vi "Periodic Tasks.vi"(8 "error in":errorcluster) -> ()   [LabVIEW 2023]
doc: "This VI runs in parallel to other tasks. It can contain as many user-defined periodic loops as you need. These can carry out PID or other sorts of timed response."
uses:
  <vilib>/Rock Robotics/WPI/DriverStation/WPI_DriverStationAllianceInfo.ctl
  ctrl defs/ctrl DRIVING FRAME selector.ctl
  ctrl defs/ctrl pivot select.ctl
  ctrl defs/ctrl driver input.ctl
  ctrl defs/ctrl FRONT FACE selector.ctl
  ctrl defs/ctrl XY coord.ctl
  ctrl defs/ctrl DRIVER target assist.ctl
  ctrl defs/ctrl LIMELIGHT STREAM selector.ctl
  ctrl defs/ctrl LIMELIGHT CAMMODE selector.ctl
  ctrl defs/ctrl LIMELIGHT LEDMODE selector.ctl
  <vilib>/Analysis/coordinate.llb/Angle Units.ctl
  <vilib>/Analysis/coordinate.llb/Angle Range (Degree).ctl
  <vilib>/Analysis/coordinate.llb/Wrap Angle (scalar).vi
  Global odometry.vi
  Global INIT.vi
  <vilib>/Analysis/NI_AAL_Angle.lvlib
panel:
  out "LimeLIGHT control":T4 {"stream" items=["standard side-by-side", "PiP Main", "PiP Secondary"]; "camMode" items=["Vision processor", "Driver Camera"]; "ledMode" items=["default to current pipeline", "force off", "force blink", "force on"]}
  out "DRIVER TARGET ASSIST":T5={"ASSIST?"=FALSE, "LOCKED ON?"=FALSE, "DistanceToTarget (in)"=26.235051697949295, "BRNG (deg)"=-2.0}
  out "Continuous Angle":T6
  in  "Update":bool
  out "pivot center":T7 {"Y" format="%.4g"; "X" format="%.4g"}
  out "front face":T8
  out "DRIVER INPUT":T9 {"Jr" format="%.4g"; "theta (rad)" format="%_4f"; "R" format="%.4g"; "Jy" format="%.4g"; "theta (deg)" format="%_4f"; "Jx" format="%.4g"}
  out "select pivot point":T10
  out "drive frame":T11
  out "Alliance":T12
  out "STEER":dbl
  out "DRIVE":dbl
  out "YRPHfH":T13
  out "REAR RIGHT":dbl(knob)
  out "V RR":dbl(knob) scale=-1.0..1.0
  out "FRONT RIGHT":dbl(knob)
  out "V FR":dbl(knob) scale=-1.0..1.0
  out "REAR LEFT":dbl(knob)
  out "V RL":dbl(knob) scale=-1.0..1.0
  out "FRONT LEFT":dbl(knob)
  out "V FL":dbl(knob) scale=-1.0..1.0
  out "Magnetic\nHeadings":cluster{dbl, dbl, dbl}(knob)={0.0, 140.19422999815168, 0.0} scale=0.0..360.0
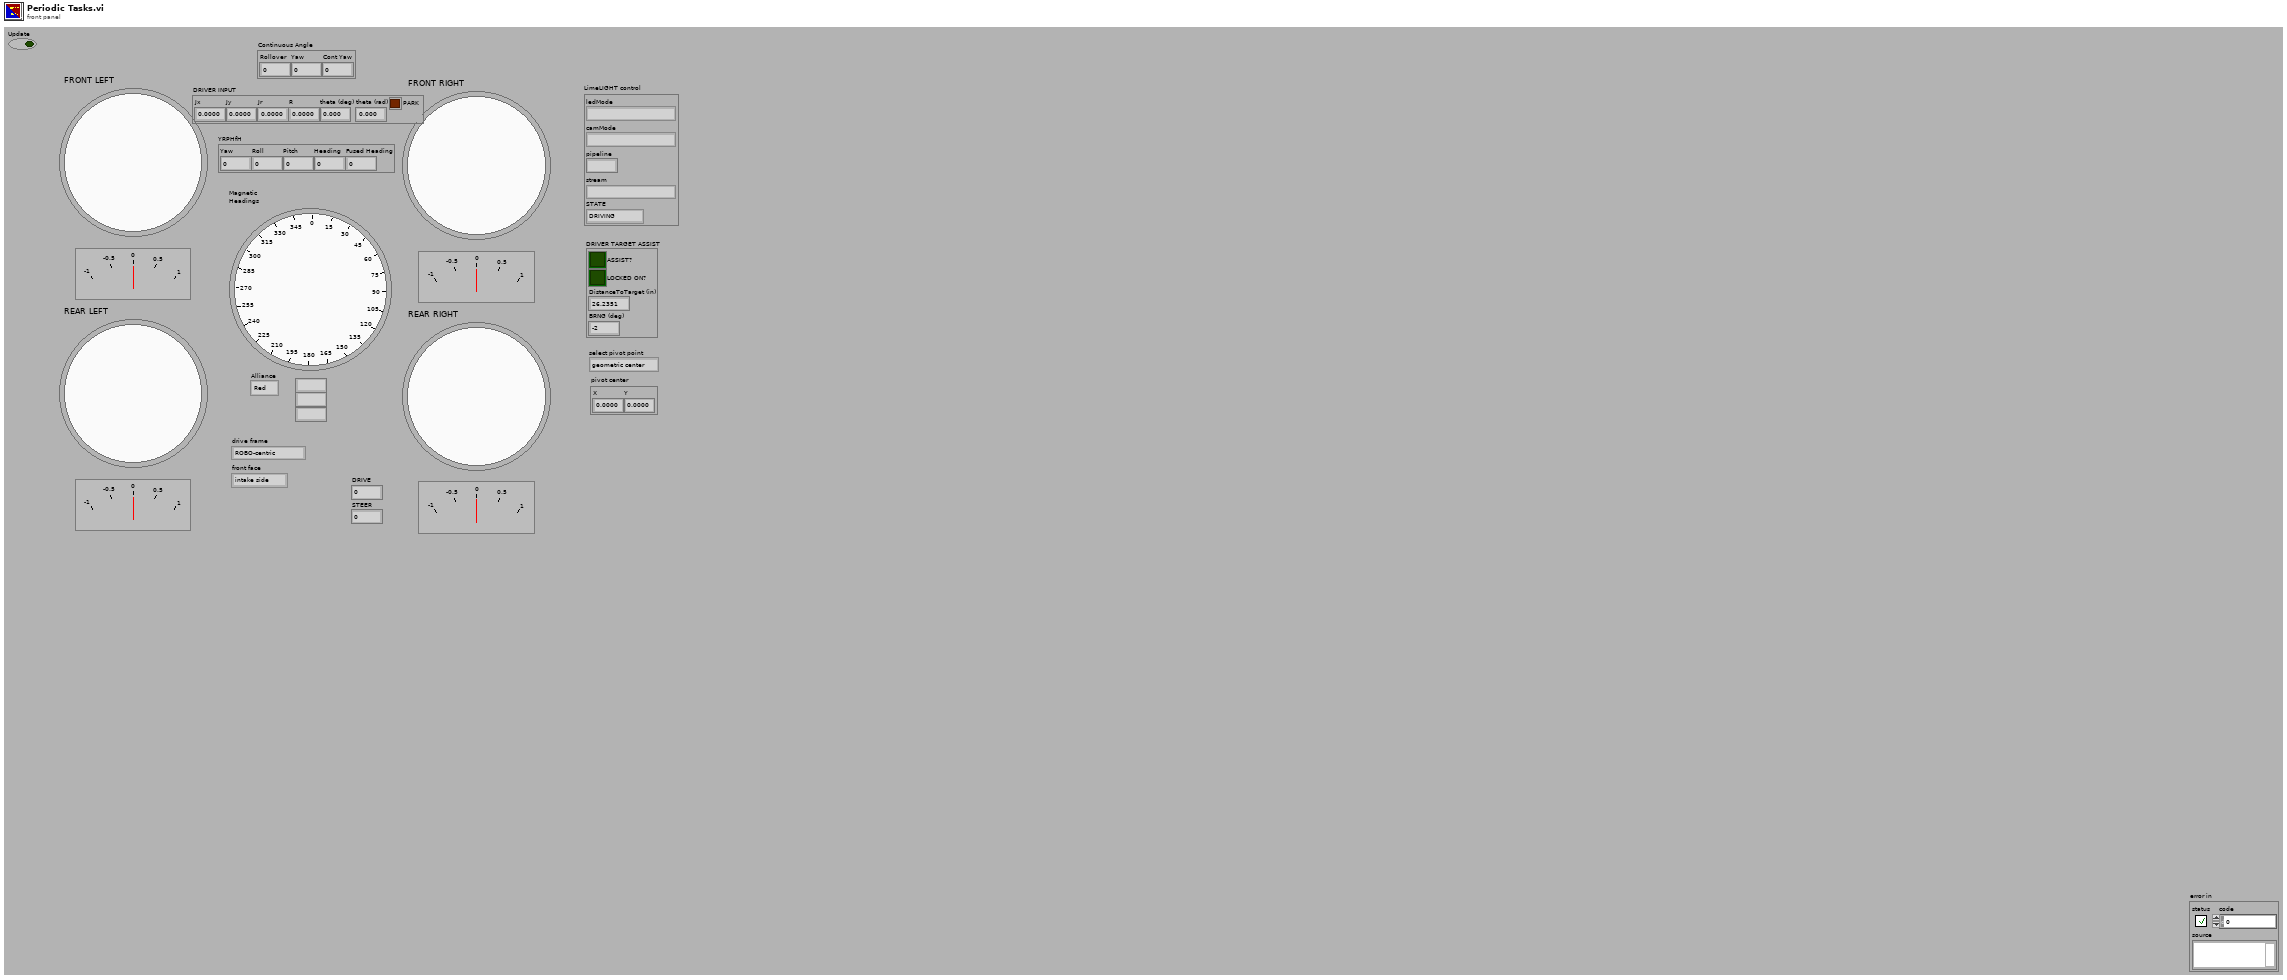
[diagram p1: front panel]
types:
  T1 = typedef "ctrl LIMELIGHT STREAM selector.ctl" = u16
  T2 = typedef "ctrl LIMELIGHT CAMMODE selector.ctl" = u16
  T3 = typedef "ctrl LIMELIGHT LEDMODE selector.ctl" = u16
  T4 = cluster{"stream":T1, "pipeline":u16, "camMode":T2, "ledMode":T3, "STATE":enum16{"DRIVING", "LOOKING for NOTE", "HAVE NOTE"}}
  T5 = typedef "ctrl DRIVER target assist.ctl" = cluster{"ASSIST?":bool, "LOCKED ON?":bool, "DistanceToTarget (in)":dbl, "BRNG (deg)":dbl}
  T6 = cluster{"Rollover":dbl, "Yaw":dbl, "Cont Yaw":dbl}
  T7 = typedef "ctrl XY coord.ctl" = cluster{"X":dbl, "Y":dbl}
  T8 = typedef "ctrl FRONT FACE selector.ctl" = enum16{"intake side", "shooter side"}
  T9 = typedef "ctrl driver input.ctl" = cluster{"Jx":dbl, "Jy":dbl, "Jr ":dbl, "R":dbl, "theta (deg)":dbl, "theta (rad)":dbl, "PARK":bool}
  T10 = typedef "ctrl pivot select.ctl" = enum16{"geometric center", "CG", "FL", "FR", "RR", "RL", "other"}
  T11 = typedef "ctrl DRIVING FRAME selector.ctl" = enum16{"ROBO-centric", "FLD-centric"}
  T12 = typedef "WPI_DriverStationAllianceInfo.ctl" = enum16{"Red", "Blue", "Invalid"}
  T13 = cluster{"Yaw":dbl, "Roll":dbl, "Pitch":dbl, "Heading":dbl, "Fused Heading":dbl}
  T14 = typedef "ctrl arm motor.ctl" = cluster{" motor":T15, "limit polarities":T21}
  T15 = typedef "ctrl swerve motor.ctl" = cluster{"description":string, "MOTOR SELECT":T16, "Installed?":bool, "CAN ID":u8, "refnum name":string, "Invert":bool, "Idle Mode":T17, "Current limiting":T18, "MOTOR PIDF coefficients":T19, "gear ratio":dbl}
  T16 = typedef "ctrl MOTOR SELECT.ctl" = i16
  T17 = typedef "Spark MAX Idle Mode.ctl" = enum16{"Coast", "Brake"}
  T18 = typedef "ctrl Spark MAX current limiting.ctl" = cluster{"Linearized":bool, "Free Speed (A)":dbl, "Primay (A)":dbl, "Limit RPM (0)":u32}
  T19 = typedef "ctrl motor PIDF coefficients.ctl" = cluster{"PIDF":cluster{"P Gain":dbl, "I Gain":dbl, "D Gain":dbl, "F Gain":dbl, "I Zone":dbl, "Min Output":dbl, "Max Output":dbl}, "Smart Motion":T20}
  T20 = typedef "Spark MAX Smart Motion Parameters.ctl" = cluster{"Max Velocity":dbl, "Max Acceleration":dbl, "Minimum Velocity Output":dbl, "Allowed Closed Loop Error":dbl}
  T21 = typedef "ctrl limit polarity.ctl" = cluster{"Forward limit":T22, "Reverse limit":T22}
  T22 = typedef "Spark MAX Limit Switch Polarity.ctl" = enum16{"Normally Open", "Normally Closed"}
  T23 = typedef "ctrl LED init.ctl" = cluster{"PWM Channel":T24, "refnum name":string, "#LEDS":T25, "initial output":dbl, "stack name":string, "Installed?":bool, "pattern":T26}
  T24 = typedef "FPGA_DIOPWMChannel.ctl" = enum8{"PWM 0", "PWM 1", "PWM 2", "PWM 3", "PWM 4", "PWM 5", "PWM 6", "PWM 7", "PWM 8", "PWM 9", "PWM MXP 0", "PWM MXP 1", "PWM MXP 2", "PWM MXP 3", "PWM MXP 4", "PWM MXP 5", "PWM MXP 6", "PWM MXP 7", "PWM MXP 8", "PWM MXP 9", "Invalid"}
  T25 = typedef "ctrl number of LEDs.ctl" = u16
  T26 = typedef "ctrl LED PATTERNS.ctl" = u16
  T27 = typedef "ctrl DIO.ctl" = cluster{"description":string, "Installed?":bool, "DIOChannel":T28, "refnum name":string}
  T28 = typedef "FPGA_DIOChannel.ctl" = enum8{"DIO 0", "DIO 1", "DIO 2", "DIO 3", "DIO 4", "DIO 5", "DIO 6", "DIO 7", "DIO 8", "DIO 9", "DIO MXP 0", "DIO MXP 1", "DIO MXP 2", "DIO MXP 3", "DIO MXP 4", "DIO MXP 5", "DIO MXP 6", "DIO MXP 7", "DIO MXP 8", "DIO MXP 9", "DIO MXP 10", "DIO MXP 11", "DIO MXP 12", "DIO MXP 13", "DIO MXP 14", "DIO MXP 15", "SPI Port CS1", "SPI Port CS2", "SPI Port CS3", "SPI Port MISO", "SPI Port MOSI", "Invalid"}
  T29 = typedef "ctrl LIMELIGHT initialize.ctl" = cluster{"Installed?":bool, "pose":cluster{"X":dbl, "Y":dbl, "Z":dbl, "angle to horizon":dbl, "tx angle offset":dbl}}
  T30 = typedef "WPI_DigitalInputDevRef.ctl" = cluster{"DevStatus":errorcluster, "DIO Channel":T28}
  T31 = typedef "ctrl swerve speeds.ctl" = cluster{"NORMAL":cluster{"DRIVE":dbl, "STEER":dbl}, "TURTLE":cluster{"DRIVE":dbl, "STEER":dbl}, "TURBO":cluster{"DRIVE":dbl, "STEER":dbl}}
  T32 = typedef "ctrl solenoid.ctl" = cluster{"description":string, "Installed?":bool, "refnum name":string, "coils":enum16{"Single", "Double"}, "forward channel":T33, "reverse channel":T33, "initial value":T34}
  T33 = typedef "WPI_SolenoidChannel.ctl" = enum8{"Solenoid 0", "Solenoid 1", "Solenoid 2", "Solenoid 3", "Solenoid 4", "Solenoid 5", "Solenoid 6", "Solenoid 7", "Solenoid 8", "Solenoid 9", "Solenoid 10", "Solenoid 11", "Solenoid 12", "Solenoid 13", "Solenoid 14", "Solenoid 15", "Invalid"}
  T34 = typedef "WPI_SolenoidValue.ctl" = enum16{"Off", "On", "Forward", "Reverse"}
  T35 = cluster{"LEFT ARM":cluster{"VBus%":dbl, "LOCK?":bool, "LOCKED":bool}, "RIGHT ARM":cluster{"VBus%":dbl, "LOCK?":bool, "LOCKED":bool}}
  T36 = cluster{"VBus%":dbl, "LOCK?":bool, "LOCKED":bool}
  T37 = typedef "WPI_MotorControlDeviceRef.ctl" = cluster{"DeviceStatus":errorcluster, "Type":T38, "PWM":cluster{"PWM Channel":T24, "DeadBand":T39}, "CAN":cluster{"Device Number":u8, "SetOutput VI Ref":variant, "GetOutput VI Ref":variant, "Enable VI Ref":variant, "Disable VI Ref":variant, "Data":variant}, "Invert":bool, "DIO PWM":cluster{"PWM \"Enable\" Channel":T24, "DIOChannel":T28, "PWM Rate":dbl}}
  T38 = typedef "WPI_MotorControlType.ctl" = enum16{"PWM", "CAN", "DIO PWM"}
  T39 = typedef "WPI_PWMDeadband.ctl" = cluster{"Name":string, "maxPositivePwm":i32, "minPositivePwm":i32, "centerPwm":i32, "maxNegativePwm":i32, "minNegativePwm":i32, "angularRange":u16}
  T40 = typedef "CTRE_Phoenix_CANcoder_DeviceRef.ctl" = cluster{"DeviceStatus":errorcluster, "Device Number":u8, "Handle":u64, "UsageFrame":u32, "Library Path":path}
  T41 = cluster{"Driver":T37, "Steer":T37, "Encoder":T40}[]
  T42 = typedef "NI_AAL_Angle.lvlib/Angle Range (Degree).ctl" = u16
  T43 = typedef "NI_AAL_Angle.lvlib/Angle Units.ctl" = i32
  T44 = cluster{"Heading":dbl, "MAGNETIC Zero for Blue Alliance (deg)":dbl, "angle out":dbl}
  T45 = typedef "ctrl DRIVER MODE.ctl" = enum16{"default", "TURTLE", "TURBO"}
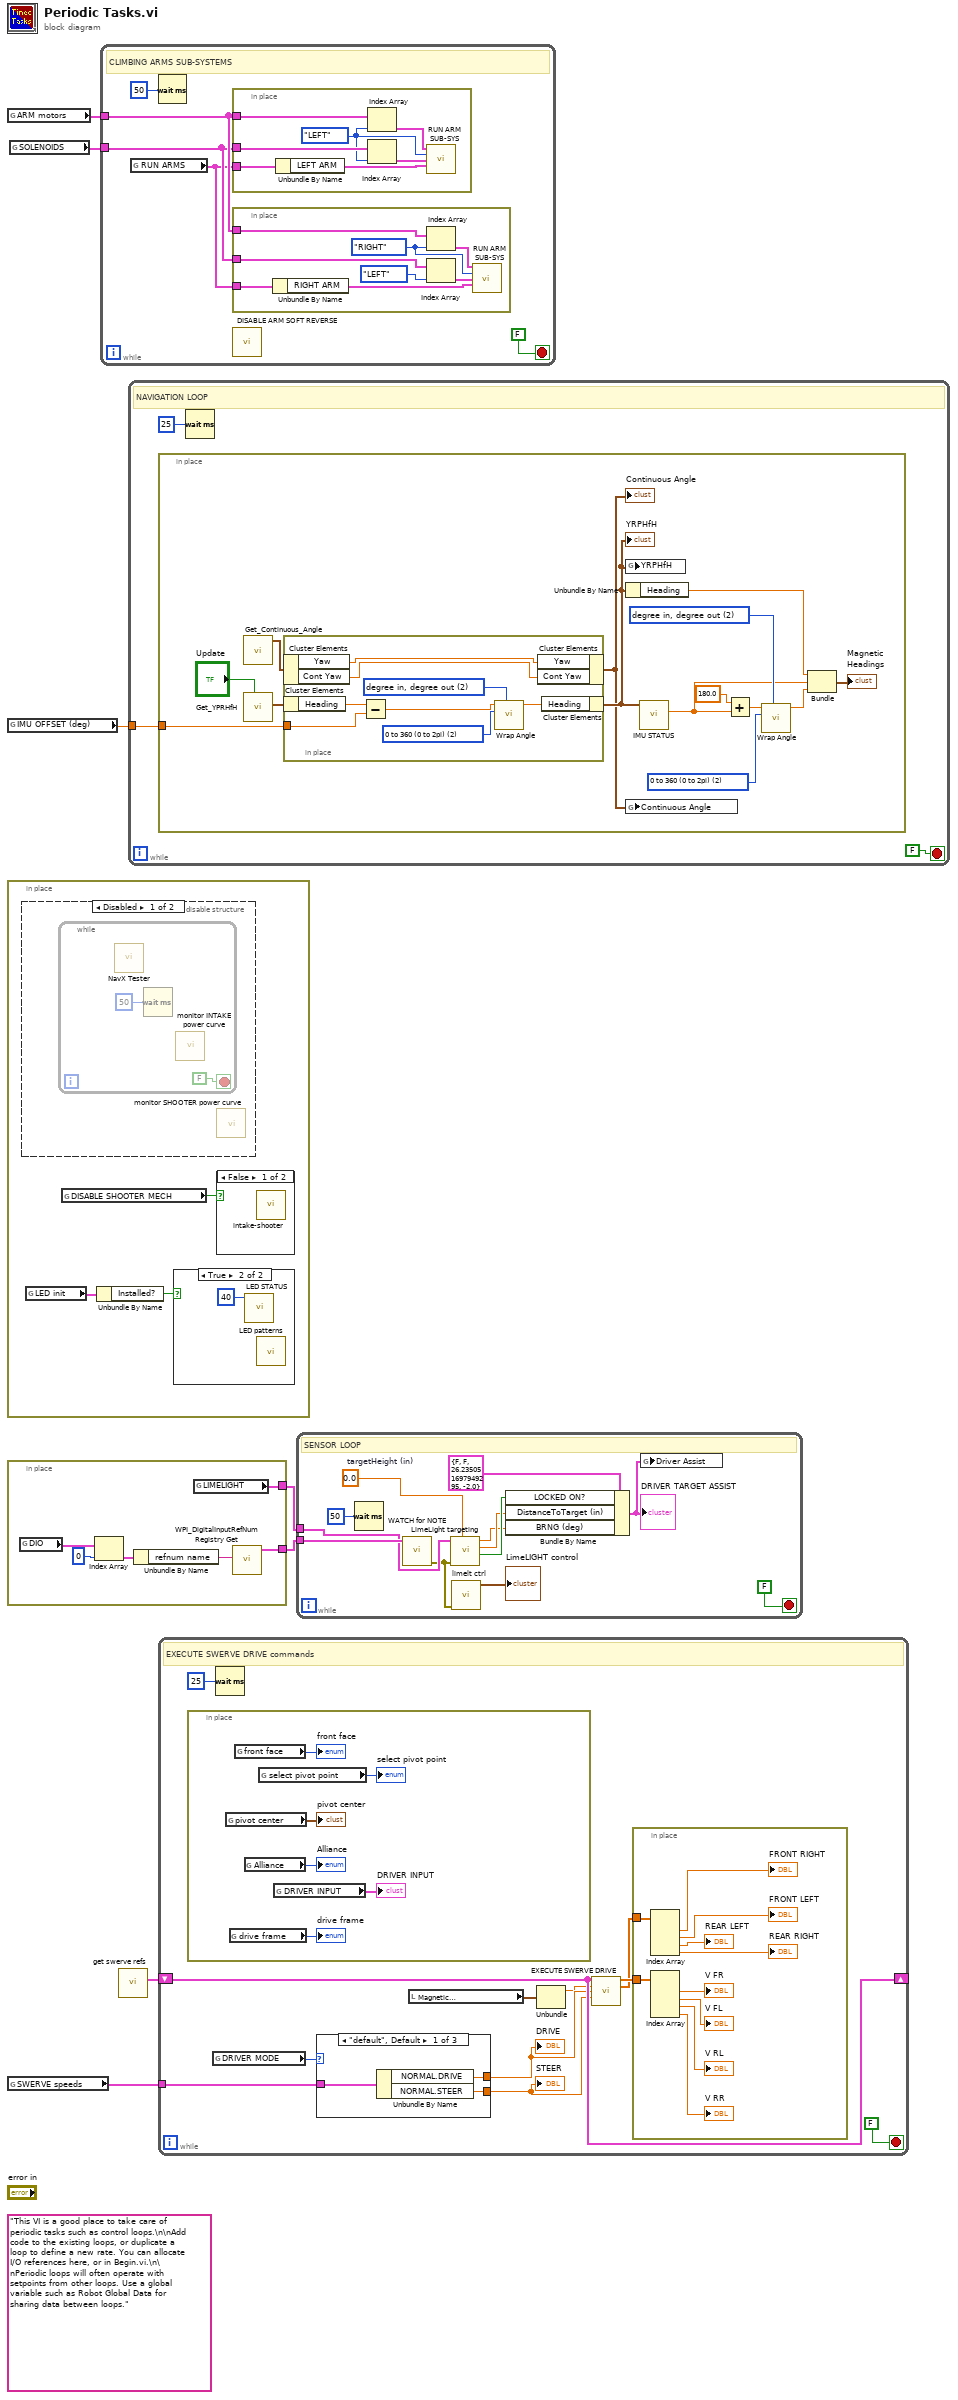
[diagram p0: block diagram]
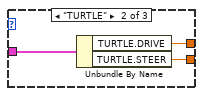
[diagram p5: hidden frame]
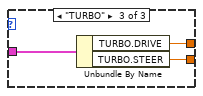
[diagram p6: hidden frame]
diagram:
  (unwired) "This VI is a good place to take care of periodic tasks such as control loops.\n\nAdd code to the existing loops, or duplicate a loop to define a new rate. You can allocate I/O references here, or in Begin.vi.\n\nPeriodic loops will often operate with setpoints from other loops. Use a global variable such as Robot Global Data for sharing data between loops."
  n1 = global read "Global INIT.vi" "ARM motors"() -> (w4:T14[])
  n2 = global read "Global INIT.vi" "IMU OFFSET (deg)"() -> (w3:dbl)
  n3 = in-place {
    n4 = disable-structure shown="Disabled" {
      frame Disabled {
        n5 = while {
          stop <- FALSE stop-if-true
          n6 = call <vilib>:"NavX Tester.vi"() -> ()  [unwired: 1 in]
          n7 = Wait (ms)(milliseconds to wait=u32 50) -> ()  [unwired: 1 out]
          n8 = call "monitor INTAKE power curve.vi"() -> ()  [unwired: 16 in]
        }
        n9 = call "monitor SHOOTER power curve.vi"() -> ()  [unwired: 16 in]
      }
      frame Enabled {
      }
    }
    n10 = global read "Global INIT.vi" "LED init"() -> (w8:T23)
    n11 = global read "Global INIT.vi" "DISABLE SHOOTER MECH"() -> (w10:bool)
    n12 = Unbundle By Name(w8) -> ("Installed?"=w9:bool)
    n13 = case shown="True" w9 {
      frame False {
      }
      frame True {
        n14 = call "LED STATUS.vi"("LOOP (ms)"=u32 40) -> ()  [unwired: 10 in, 1 out]
        n15 = call "LED patterns.vi"() -> ()  [unwired: 12 in]
      }
    }
    n16 = case shown="False" w10 {
      frame False {
        n17 = call "intake-shooter.vi"() -> ()  [unwired: 12 in]
      }
      frame True {
      }
    }
  }
  n18 = in-place {
    in-place-border: [w15] -> w2
    in-place-border: [w14] -> w1
    n19 = global read "Global INIT.vi" "DIO"() -> (w19:T27[])
    n20 = Index Array(array=w19, index=0) -> (element=w17:T27)
    n21 = Unbundle By Name(w17) -> ("refnum name"=w16:string)
    n22 = global read "Global INIT.vi" "LIMELIGHT"() -> (w14:T29)
    n23 = call <vilib>:"WPI_DigitalInputRefNum Registry Get.vi"("refnum name"=w16) -> ("DigitalInputDevRef"=w15:T30)  [unwired: 9 in, 1 out]
  }
  n24 = global read "Global odometry.vi" "SWERVE speeds"() -> (w6:T31)
  n25 = global read "Global INIT.vi" "SOLENOIDS"() -> (w5:T32[])
  n26 = while {
    tunnel: w5 -> [w21]
    tunnel: w4 -> [w22]
    stop <- FALSE stop-if-true
    # "CLIMBING ARMS SUB-SYSTEMS"
    n27 = global read "Global odometry.vi" "RUN ARMS"() -> (w20:T35)
    n28 = Wait (ms)(milliseconds to wait=u32 50) -> ()  [unwired: 1 out]
    n29 = in-place {
      in-place-border: w22 -> [w38]
      in-place-border: w21 -> [w36]
      in-place-border: w20 -> [w35]
      w34 = enum16{"LEFT", "RIGHT"}."LEFT" ("SIDE")
      n30 = Unbundle By Name(w35) -> ("LEFT ARM"=w39:T36)
      n31 = Index Array(array=w38, index=w34) -> (element=w37:T14)
      n32 = Index Array(array=w36, index=w34) -> (element=w33:T32)
      n33 = call "RUN ARM SUB-SYS.vi"("ARM motor"=w37, "SIDE"=w34, "SOLENOID"=w33, "ARM"=w39) -> ()  [unwired: 12 in]
    }
    n34 = in-place {
      in-place-border: w22 -> [w31]
      in-place-border: w21 -> [w29]
      in-place-border: w20 -> [w28]
      w27 = enum16{"LEFT", "RIGHT"}."RIGHT" ("SIDE")
      n35 = Unbundle By Name(w28) -> ("RIGHT ARM"=w32:T36)
      n36 = Index Array(array=w31, index=w27) -> (element=w30:T14)
      n37 = Index Array(array=w29, index=enum16{"LEFT", "RIGHT"}."LEFT" ("SIDE")) -> (element=w26:T32)
      n38 = call "RUN ARM SUB-SYS.vi"("ARM motor"=w30, "SIDE"=w27, "SOLENOID"=w26, "ARM"=w32) -> ()  [unwired: 12 in]
    }
    n39 = call "DISABLE ARM SOFT REVERSE.vi"() -> ()  [unwired: 12 in]
  }
  n40 = call "get swerve refs.vi"() -> ("Swerve refs"=w7:T41)  [unwired: 10 in, 1 out]
  n41 = while {
    tunnel: w3 -> [w40]
    stop <- FALSE stop-if-true
    # "NAVIGATION LOOP"
    n42 = in-place {
      in-place-border: w40 -> [w47]
      w53 = T42 2 items=["none", "-180 to 180 (-pi to pi)", "0 to 360 (0 to 2pi)"] ("angle range")
      w54 = T43 2 items=["radian in, radian out", "radian in, degree out", "degree in, degree out", "degree in, radian out"] ("angle units")
      n43 = call <vilib>:"Get_Continuous_Angle.vi"() -> ("Continuous Angle"=w44:T6)  [unwired: 11 in]
      n44 = call <vilib>:"Get_YPRHfH.vi"("Update"="Update") -> ("YRPHfH"=w48:T13)  [unwired: 10 in]
      n45 = in-place {
        in-place-border: w47 -> [w59]
        w60 = T42 2 items=["none", "-180 to 180 (-pi to pi)", "0 to 360 (0 to 2pi)"] ("angle range")
        w61 = T43 2 items=["radian in, radian out", "radian in, degree out", "degree in, degree out", "degree in, radian out"] ("angle units")
        n46 = in-place-cluster #1(w44) -> ("Yaw"=w58:dbl, "Cont Yaw"=w57:dbl)
        n47 = in-place-cluster #2(w48) -> ("Heading"=w64:dbl)
        n48 = Subtract(x=w64, y=w59) -> (x-y=w63:dbl)
        n49 = call-poly <vilib>:"Wrap Angle.vi"("angle units"=w61, "angle range"=w60, "angle in"=w63) -> ("angle out"=w62:dbl)  [unwired: 7 in, 1 out]
        n50 = in-place-cluster #1("Yaw"=w58, "Cont Yaw"=w57) -> (w43:T6)
        n51 = in-place-cluster #2("Heading"=w62) -> (w45:T13)
      }
      "YRPHfH" <- w45
      "Continuous Angle" <- w43
      n52 = global write "Global odometry.vi" "YRPHfH"(w45) -> ()
      n53 = Unbundle By Name(w45) -> ("Heading"=w56:dbl)
      n54 = global write "Global odometry.vi" "Continuous Angle"(w43) -> ()
      n55 = call "IMU STATUS.vi"("YRPHfH"=w45) -> ("MAGNETIC Zero for Blue Alliance (deg)"=w51:dbl)  [unwired: 9 in, 1 out]
      n56 = Add(x=180.0, y=w51) -> (x+y=w50:dbl)
      n57 = call-poly <vilib>:"Wrap Angle.vi"("angle units"=w54, "angle range"=w53, "angle in"=w50) -> ("angle out"=w52:dbl)  [unwired: 7 in, 1 out]
      n58 = Bundle("Heading"=w56, "MAGNETIC Zero for Blue Alliance (deg)"=w51, "angle out"=w52) -> (→"Magnetic\nHeadings":T44)  [unwired: 1 in]
    }
    n59 = Wait (ms)(milliseconds to wait=u32 25) -> ()  [unwired: 1 out]
  }
  n60 = while {
    shift-right: [w72] -> _
    shift-left: w7 -> [w72]
    tunnel: w6 -> [w73]
    stop <- FALSE stop-if-true
    # "EXECUTE SWERVE DRIVE commands"
    n61 = in-place {
      n62 = global read "Global odometry.vi" "pivot center"() -> (→"pivot center":T7)
      n63 = global read "Global odometry.vi" "drive frame"() -> (→"drive frame":T11)
      n64 = global read "Global odometry.vi" "front face"() -> (→"front face":T8)
      n65 = global read "Global odometry.vi" "Alliance"() -> (→"Alliance":T12)
      n66 = global read "Global odometry.vi" "select pivot point"() -> (→"select pivot point":T10)
      n67 = global read "Global odometry.vi" "DRIVER INPUT"() -> (→"DRIVER INPUT":T9)
    }
    n68 = global read "Global odometry.vi" "DRIVER MODE"() -> (w71:T45)
    n69 = Wait (ms)(milliseconds to wait=u32 25) -> ()  [unwired: 1 out]
    n70 = case shown="\"default\", Default" w71 {
      tunnel: w73 -> [w93 w97 w99]
      tunnel: [w94 w96 w100] -> w70
      tunnel: [w92 w95 w98] -> w69
      frame "default", Default {
        n71 = Unbundle By Name(w93) -> ("NORMAL.DRIVE"=w94:dbl, "NORMAL.STEER"=w92:dbl)
      }
      frame "TURTLE" {
        n72 = Unbundle By Name(w97) -> ("TURTLE.DRIVE"=w96:dbl, "TURTLE.STEER"=w95:dbl)
      }
      frame "TURBO" {
        n73 = Unbundle By Name(w99) -> ("TURBO.DRIVE"=w100:dbl, "TURBO.STEER"=w98:dbl)
      }
    }
    "DRIVE" <- w70
    "STEER" <- w69
    n74 = local read "Magnetic\nHeadings"() -> (w68:cluster{dbl, dbl, dbl})
    n75 = Unbundle(w68) -> (w67:dbl)  [unwired: 2 out]
    n76 = call "EXECUTE SWERVE DRIVE.vi"("Swerve refs"=w72, "HEADING"=w67, "DRIVE MAX SPEED"=w70, "STEER MAX speed"=w69) -> ("VELOCITIES"=w66:dbl[], "STEERING\nANGLES (deg)"=w65:dbl[])  [unwired: 10 in]
    n77 = in-place {
      in-place-border: w66 -> [w91]
      in-place-border: w65 -> [w86]
      n78 = Index Array(array=w86) -> (element #1=→"FRONT RIGHT":dbl, element #2=→"FRONT LEFT":dbl, element #3=→"REAR LEFT":dbl, element #4=→"REAR RIGHT":dbl)  [unwired: 4 in]
      n79 = Index Array(array=w91) -> (element #1=→"V FR":dbl, element #2=→"V FL":dbl, element #3=→"V RL":dbl, element #4=→"V RR":dbl)  [unwired: 4 in]
    }
  }
  n80 = while {
    tunnel: w2 -> [w112]
    tunnel: w1 -> [w109]
    stop <- FALSE stop-if-true
    w108 = 0.0  # targetHeight (in)
    # "SENSOR LOOP"
    n81 = Wait (ms)(milliseconds to wait=u32 50) -> ()  [unwired: 1 out]
    n82 = call "WATCH for NOTE.vi"("DigitalInputDevRef"=w112) -> ("error out"=w102:errorcluster)  [unwired: 10 in]
    n83 = call "LimeLight targeting.vi"("targetHeight (in)"=w108, "error in (no error)"=w102, "LIMELIGHT pose"=w109) -> ("LOCK?"=w105:bool, "DistanceToTarget"=w104:dbl, "BRNG (deg)"=w103:dbl)  [unwired: 5 in, 1 out]
    n84 = call "limelt ctrl.vi"("error in (no error)"=w102) -> ("LimeLIGHT control"=→"LimeLIGHT control":T4)  [unwired: 9 in, 1 out]
    n85 = Bundle By Name(cluster=T5 {"ASSIST?"=FALSE, "LOCKED ON?"=FALSE, "DistanceToTarget (in)"=26.235051697949295, "BRNG (deg)"=-2.0} ("Driver Assist"), "LOCKED ON?"=w105, "DistanceToTarget (in)"=w104, "BRNG (deg)"=w103) -> (w106:T5)
    "DRIVER TARGET ASSIST" <- w106
    n86 = global write "Global odometry.vi" "Driver Assist"(w106) -> ()
  }
